vi "Digital Output 0-10V.vi"(8 "error in (no error)":errorcluster, 9 "State":bool, 10 "#Pin 0-10V":enum16{"DO-0", "DO-1", "DO-2", "DO-3"}(ring), 11 "Modbus Master in":refnum<class "Modbus Master.lvclass">) -> (0 "error out":errorcluster, 2 "State Send?":bool, 3 "Modbus master out":refnum<class "Modbus Master.lvclass">)   [LabVIEW 2020, in "Hardware DAQ.lvlib"]
uses:
  Hardware DAQ.lvlib
  <vilib>/Modbus/master/Modbus Master.lvclass
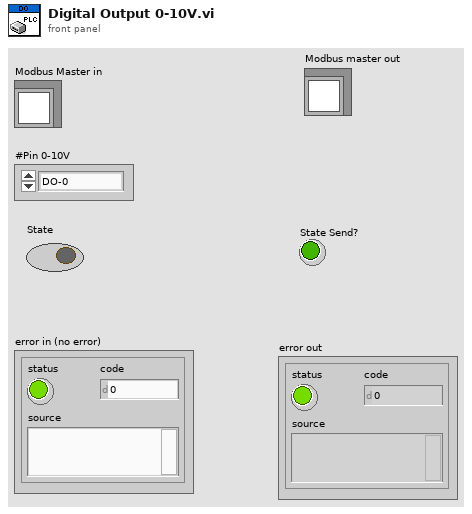
[diagram p1: front panel]
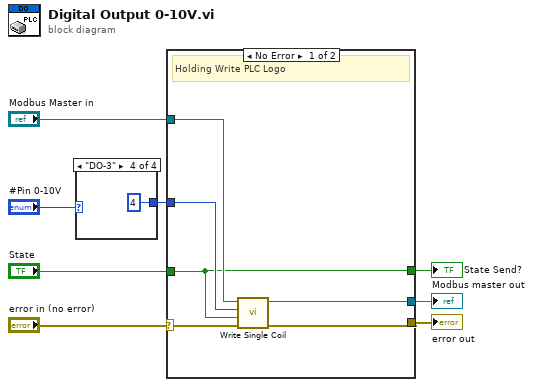
[diagram p0: block diagram]
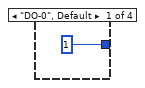
[diagram p2: hidden frame]
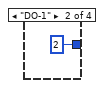
[diagram p3: hidden frame]
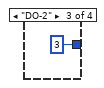
[diagram p4: hidden frame]
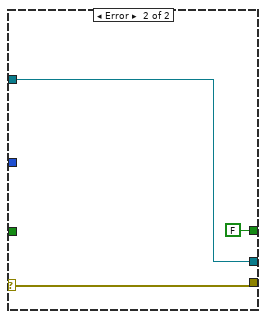
[diagram p5: hidden frame]
diagram:
  n1 = case shown="\"DO-3\"" "#Pin 0-10V" {
    tunnel: [u16 1 ("address") u16 2 ("address") u16 3 ("address") u16 4 ("address")] -> w4
    frame "DO-0", Default {
    }
    frame "DO-1" {
    }
    frame "DO-2" {
    }
    frame "DO-3" {
    }
  }
  n2 = case shown="No Error" "error in (no error)" {
    selector: "error in (no error)" -> [w18 w21]
    tunnel: "Modbus Master in" -> [w16 w20]
    tunnel: [w17 w21] -> w2
    tunnel: "State" -> [w13 _]
    tunnel: w4 -> [w15 _]
    tunnel: [w14 w20] -> w3
    tunnel: [w13 FALSE ("State")] -> w1
    frame No Error {
      # "Holding Write PLC Logo"
      n3 = call-dynamic "Write Single Coil.vi"("error in (no error)"=w18, "coil value"=w13, "address"=w15, "Modbus master in"=w16) -> ("error out"=w17:errorcluster, "Modbus master out"=w14:refnum<class "Modbus Master.lvclass">)  [unwired: 6 in]
    }
    frame Error {
    }
  }
  "Modbus master out" <- w3
  "error out" <- w2
  "State Send?" <- w1
